vi "0-99 NUMBER TO STRING(SubVI).vi"(1 "A":dbl) -> (0 "element":string)   [LabVIEW 2019]
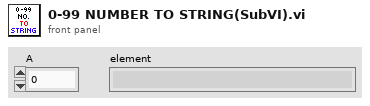
[diagram p1: front panel]
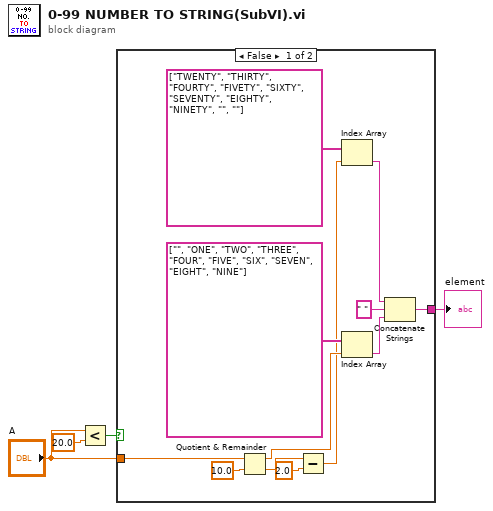
[diagram p0: block diagram]
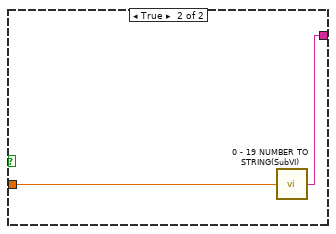
[diagram p2: hidden frame]
diagram:
  n1 = Less?(x="A", y=20.0) -> (x < y?=w2:bool)
  n2 = case shown="False" w2 {
    tunnel: "A" -> [w16 w18]
    tunnel: [w5 w17] -> w4
    frame False {
      n3 = Quotient & Remainder(x=w16, y=10.0) -> (x-y*floor(x/y)=w13:dbl, floor(x/y)=w12:dbl)
      n4 = Subtract(x=w12, y=2.0) -> (x-y=w10:dbl)
      n5 = Index Array(array=string[] ["TWENTY", "THIRTY", "FOURTY", "FIVETY", "SIXTY", "SEVENTY", "EIGHTY", "NINETY", "", ""], index=w10) -> (element=w8:string)
      n6 = Index Array(array=string[] ["", "ONE", "TWO", "THREE", "FOUR", "FIVE", "SIX", "SEVEN", "EIGHT", "NINE"], index=w13) -> (element=w7:string)
      n7 = Concatenate Strings(w8, " " ("string"), w7) -> (w5:string)
    }
    frame True {
      n8 = call "0 - 19 NUMBER TO STRING(SubVI).vi"("A"=w18) -> ("element"=w17:string)
    }
  }
  "element" <- w4
